vi "DHE_Utils.vi"(0 "refnum":i32, 5 "Command":string, 7 "physical unit":string, 11 "error in (no error)":errorcluster) -> (4 "refnum out":i32, 6 "message":string, 8 "Read Value":i32, 15 "error out":errorcluster)   [LabVIEW 2016]
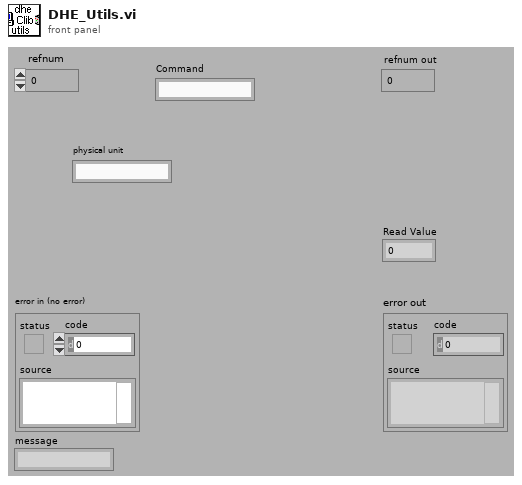
[diagram p1: front panel]
types:
  T1 = typedef "CMN_ContStatus.ctl" = cluster{"Response":string, "power":bool, "shutter":bool, "artifdata":bool, "idlemode":bool, "reset":bool, "gain":u8, "speed":u8, "resetPCI":bool, "autoshutter":bool, "TempSetPoint":i32, "multipleextensions":bool, "displayImage":bool, "coadding":bool, "images being coadded":i32, "Operation Mode":enum16{"normal", "coadd", "fawler"}, "frames to write":cluster{"subs":bool, "reset":bool, "exposed":bool}, "fawler samples":i32, "write auto":bool, "datatype":string, "frames to display":cluster{"subs":bool, "reset":bool, "exposed":bool}, "sur":i32, "autoclear":bool}
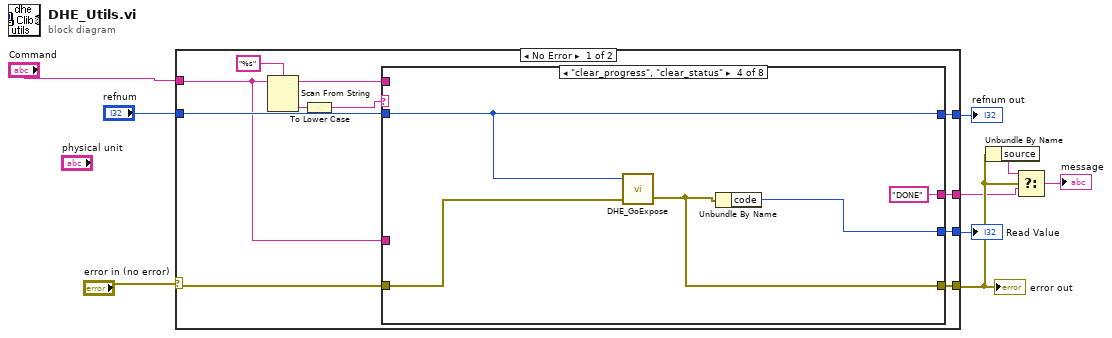
[diagram p0: block diagram]
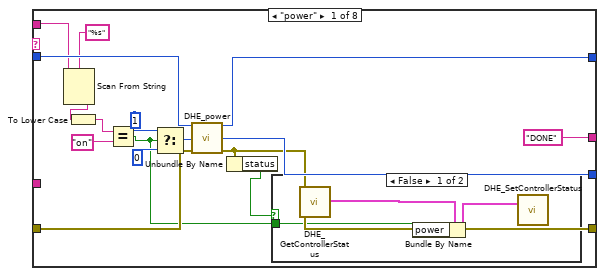
[diagram p2: hidden frame]
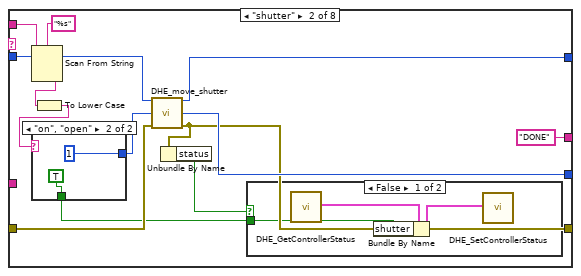
[diagram p4: hidden frame]
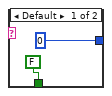
[diagram p5: hidden frame]
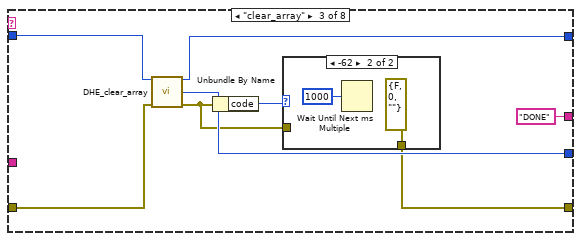
[diagram p7: hidden frame]
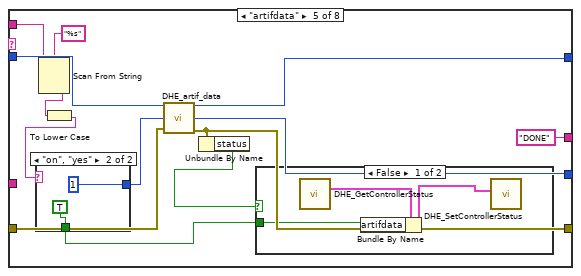
[diagram p9: hidden frame]
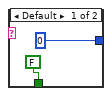
[diagram p10: hidden frame]
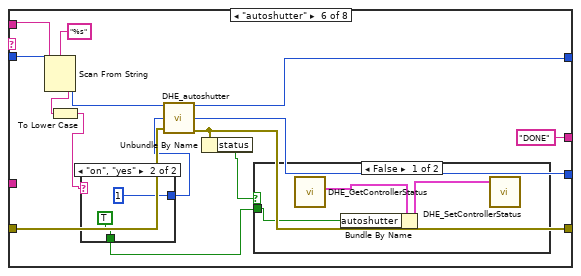
[diagram p12: hidden frame]
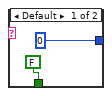
[diagram p13: hidden frame]
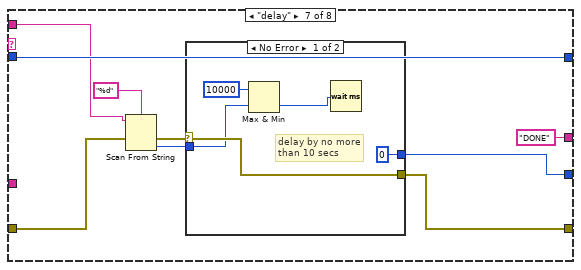
[diagram p15: hidden frame]
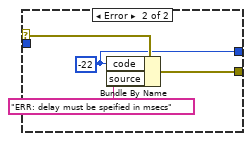
[diagram p16: hidden frame]
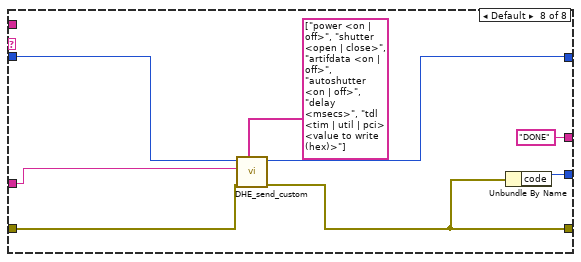
[diagram p17: hidden frame]
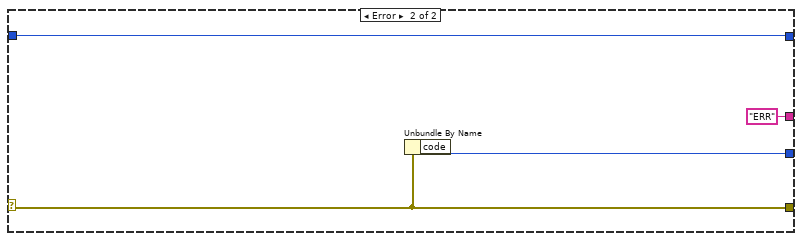
[diagram p18: hidden frame]
diagram:
  n1 = case shown="No Error" "error in (no error)" {
    selector: "error in (no error)" -> [w11 w143]
    tunnel: [w14 w143] -> w4
    tunnel: "refnum" -> [w20 w145]
    tunnel: [w19 w145] -> w8
    tunnel: "Command" -> [w12 _]
    tunnel: [w18 w144] -> w9
    tunnel: [w10 "ERR" ("message")] -> w2
    frame No Error {
      n2 = Scan From String(format string="%s" ("Format String"), input string=w12) -> (remaining string=w15:string, output 1=w16:string)  [unwired: 2 in, 3 out]
      n3 = To Lower Case(string=w16) -> (all lower case string=w13:string)
      n4 = case shown="\"clear_progress\", \"clear_status\"" w13 {
        tunnel: w11 -> [w35 w51 w66 w74 w85 w105 w121 w141]
        tunnel: w20 -> [w36 w52 w67 w75 w87 w107 w124 w137]
        tunnel: [w34 w50 w65 w75 w88 w108 w124 w136] -> w19
        tunnel: [w33 w49 w64 w72 w86 w106 w118 w140] -> w18
        tunnel: w15 -> [w26 w48 _ _ w82 w102 w123 _]
        tunnel: [w24 w45 w60 w73 w81 w101 w119 w135] -> w14
        tunnel: w12 -> [_ _ _ _ _ _ _ w134]
        tunnel: ["DONE" "DONE" "DONE" "DONE" ("message") "DONE" "DONE" "DONE" ("message") "DONE" ("message")] -> w10
        frame "power" {
          n5 = Scan From String(format string="%s" ("Format String"), input string=w26) -> (output 1=w28:string)  [unwired: 2 in, 4 out]
          n6 = To Lower Case(string=w28) -> (all lower case string=w27:string)
          n7 = Equal?(x=w27, y="on") -> (x = y?=w22:bool)
          n8 = Select(t=1, s=w22, f=0) -> (s? t:f=w30:i32)
          n9 = call "DHE_power.vi"("fd"=w36, "flag"=w30, "error in (no error)"=w35) -> ("fd out"=w34:i32, "return value"=w33:i32, "error out"=w24:errorcluster)  [unwired: 10 out]
          n10 = Unbundle By Name(w24) -> ("status"=w23:bool)
          n11 = case shown="False" w23 {
            tunnel: w22 -> [w39 _]
            frame False {
              n12 = call "DHE_GetControllerStatus.vi"() -> ("ControllerStatus"=w37:T1)  [unwired: 11 out]
              n13 = Bundle By Name(cluster=w37, "power"=w39) -> (w38:T1)
              n14 = call "DHE_SetControllerStatus.vi"("ControllerStatus"=w38) -> ()  [unwired: 1 in, 10 out]
            }
            frame True {
            }
          }
        }
        frame "shutter" {
          n15 = Scan From String(format string="%s" ("Format String"), input string=w48) -> (output 1=w46:string)  [unwired: 2 in, 4 out]
          n16 = To Lower Case(string=w46) -> (all lower case string=w43:string)
          n17 = case shown="\"on\", \"open\"" w43 {
            tunnel: [0 1] -> w42
            tunnel: [FALSE TRUE] -> w41
            frame Default {
            }
            frame "on", "open" {
            }
          }
          n18 = call "DHE_move_shutter.vi"("fd"=w52, "flag"=w42, "error in (no error)"=w51) -> ("fd out"=w50:i32, "return value"=w49:i32, "error out"=w45:errorcluster)  [unwired: 10 out]
          n19 = Unbundle By Name(w45) -> ("status"=w44:bool)
          n20 = case shown="False" w44 {
            tunnel: w41 -> [w59 _]
            frame False {
              n21 = call "DHE_GetControllerStatus.vi"() -> ("ControllerStatus"=w58:T1)  [unwired: 11 out]
              n22 = Bundle By Name(cluster=w58, "shutter"=w59) -> (w57:T1)
              n23 = call "DHE_SetControllerStatus.vi"("ControllerStatus"=w57) -> ()  [unwired: 1 in, 10 out]
            }
            frame True {
            }
          }
        }
        frame "clear_array" {
          n24 = call "DHE_clear_array.vi"("fd"=w67, "error in (no error)"=w66) -> ("fd out"=w65:i32, "return value"=w64:i32, "error out"=w61:errorcluster)  [unwired: 11 out]
          n25 = Unbundle By Name(w61) -> ("code"=w62:i32)
          n26 = case shown="-62" w62 {
            tunnel: w61 -> [w68 _]
            tunnel: [w68 errorcluster {"status"=FALSE, "code"=0, "source"=""} ("error out")] -> w60
            frame Default {
            }
            frame -62 {
              n27 = Wait Until Next ms Multiple(millisecond multiple=u32 1000) -> ()  [unwired: 1 out]
            }
          }
        }
        frame "clear_progress", "clear_status" {
          n28 = call "DHE_GoExpose.vi"("error in"=w74, "fd"=w75) -> ("error out"=w73:errorcluster)  [unwired: 2 out]
          n29 = Unbundle By Name(w73) -> ("code"=w72:i32)
        }
        frame "artifdata" {
          n30 = Scan From String(format string="%s" ("Format String"), input string=w82) -> (output 1=w83:string)  [unwired: 2 in, 4 out]
          n31 = To Lower Case(string=w83) -> (all lower case string=w78:string)
          n32 = case shown="\"on\", \"yes\"" w78 {
            tunnel: [0 1] -> w77
            tunnel: [FALSE TRUE] -> w79
            frame Default {
            }
            frame "on", "yes" {
            }
          }
          n33 = call "DHE_artif_data.vi"("fd"=w87, "flag"=w77, "error in (no error)"=w85) -> ("fd out"=w88:i32, "return value"=w86:i32, "error out"=w81:errorcluster)  [unwired: 10 out]
          n34 = Unbundle By Name(w81) -> ("status"=w80:bool)
          n35 = case shown="False" w80 {
            tunnel: w79 -> [w95 _]
            frame False {
              n36 = call "DHE_GetControllerStatus.vi"() -> ("ControllerStatus"=w94:T1)  [unwired: 11 out]
              n37 = Bundle By Name(cluster=w94, "artifdata"=w95) -> (w93:T1)
              n38 = call "DHE_SetControllerStatus.vi"("ControllerStatus"=w93) -> ()  [unwired: 1 in, 10 out]
            }
            frame True {
            }
          }
        }
        frame "autoshutter" {
          n39 = Scan From String(format string="%s" ("Format String"), input string=w102) -> (output 1=w103:string)  [unwired: 2 in, 4 out]
          n40 = To Lower Case(string=w103) -> (all lower case string=w97:string)
          n41 = case shown="\"on\", \"yes\"" w97 {
            tunnel: [0 1] -> w98
            tunnel: [FALSE TRUE] -> w99
            frame Default {
            }
            frame "on", "yes" {
            }
          }
          n42 = call "DHE_autoshutter.vi"("fd"=w107, "flag"=w98, "error in (no error)"=w105) -> ("fd out"=w108:i32, "return value"=w106:i32, "error out"=w101:errorcluster)  [unwired: 10 out]
          n43 = Unbundle By Name(w101) -> ("status"=w100:bool)
          n44 = case shown="False" w100 {
            tunnel: w99 -> [w115 _]
            frame False {
              n45 = call "DHE_GetControllerStatus.vi"() -> ("ControllerStatus"=w114:T1)  [unwired: 11 out]
              n46 = Bundle By Name(cluster=w114, "autoshutter"=w115) -> (w113:T1)
              n47 = call "DHE_SetControllerStatus.vi"("ControllerStatus"=w113) -> ()  [unwired: 1 in, 10 out]
            }
            frame True {
            }
          }
        }
        frame "delay" {
          n48 = Scan From String(format string="%d", input string=w123, error in=w121) -> (error out=w120:errorcluster, output 1=w117:i32)  [unwired: 1 in, 3 out]
          n49 = case shown="No Error" w120 {
            selector: w120 -> [w128 w133]
            tunnel: [w128 w131] -> w119
            tunnel: [0 ("code") w130] -> w118
            tunnel: w117 -> [w127 _]
            frame No Error {
              # "delay by no more \nthan 10 secs"
              n50 = Max & Min(x=10000, y=w127) -> (min(x,y)=w125:i32)  [unwired: 1 out]
              n51 = Wait (ms)(milliseconds to wait=w125) -> ()  [unwired: 1 out]
            }
            frame Error {
              w130 = -22 ("code")
              n52 = Bundle By Name(cluster=w133, "code"=w130, "source"="ERR: delay must be speified in msecs") -> (w131:errorcluster)
            }
          }
        }
        frame Default {
          n53 = call "DHE_send_custom.vi"("valid params"=string[] ["power <on | off>", "shutter <open | close>", "artifdata <on | off>", "autoshutter <on | off>", "delay <msecs>", "tdl <tim | util | pci> <value to write (hex)>"], "error in (no error)"=w141, "args"=w134, "fd"=w137) -> ("error IO"=w135:errorcluster, "fd out"=w136:i32)  [unwired: 6 out]
          n54 = Unbundle By Name(w135) -> ("code"=w140:i32)
        }
      }
    }
    frame Error {
      n55 = Unbundle By Name(w143) -> ("code"=w144:i32)
    }
  }
  "Read Value" <- w9
  "refnum out" <- w8
  "error out" <- w4
  n56 = Unbundle By Name(w4) -> ("source"=w3:string)
  n57 = Select(t=w3, s=w4, f=w2) -> (s? t:f=→"message":string)
